vi "Timeout Check.vi"(8 "Error In":errorcluster) -> (0 "Error Out":errorcluster, 3 "Still there?":bool)   [LabVIEW 2020]
uses:
  Collection Support/Controls/FirstCall.ctl
panel:
  out "Time Left":dbl format="%#.0f"
  in  "Yes!":bool
  # "Are you still there?"
  # "The program will close in"
  # "seconds"
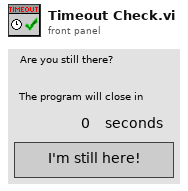
[diagram p1: front panel]
types:
  T1 = typedef "FirstCall.ctl" = enum16{"First", "After"}
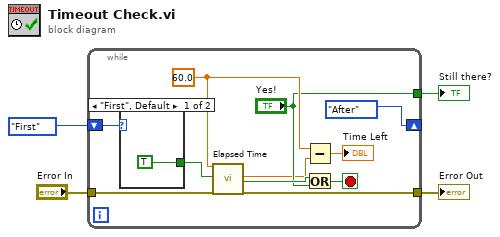
[diagram p0: block diagram]
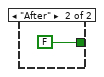
[diagram p2: hidden frame]
diagram:
  n1 = while {
    tunnel: ["Yes!"] -> w4
    tunnel: "Error In" -> [w13]
    tunnel: [w12] -> w2
    shift-right: [FirstCall."After" ("Enum")] -> _
    shift-left: FirstCall."First" ("Enum") -> [w7]
    stop <- w9 stop-if-true
    w15 = 60.0 ("Time Target (s)")
    n2 = case shown="\"First\", Default" w7 {
      tunnel: [TRUE FALSE] -> w6
      frame "First", Default {
      }
      frame "After" {
      }
    }
    n3 = call "Elapsed Time"("Time Target (s)"=w15, "Reset"=w6, "error in (no error)"=w13) -> ("Elapsed Time (s)"=w8:dbl, "Time has Elapsed"=w11:bool, "error out"=w12:errorcluster)  [unwired: 9 in, 5 out]
    n4 = Subtract(x=w15, y=w8) -> (x-y=→"Time Left":dbl)
    n5 = Or(x=w11, y="Yes!") -> (x .or. y?=w9:bool)
  }
  "Still there?" <- w4
  "Error Out" <- w2
